vi "Test_sqlite3QueriesWithNoDatabase_ReturnsError.vi"(8 "error in (no error)":errorcluster, 11 "TestCase in":refnum<class "Test sqlite3.lvclass">) -> (0 "error out":errorcluster, 3 "TestCase out":refnum<class "Test sqlite3.lvclass">)   [LabVIEW 2020, in "Test sqlite3.lvclass"]
uses:
  Test sqlite3.lvclass
  externals/sqlite3/Source/sqlite3.lvclass
  09da7179-2a0d-49b1-a176-e0431276ce58.vi
  <vilib>/Utility/error.llb/Error Cluster From Error Code.vi
  <vilib>/addons/_JKI Toolkits/VI Tester/TestCase.llb/TestCase.lvclass
  externals/database-interface/IDatabase/IDatabase/IDatabase.lvclass
  C:/Program Files/National Instruments/LabVIEW 2020/vi.lib/addons/_JKI Toolkits/VI Tester/TestCase.llb/TestCase.lvclass
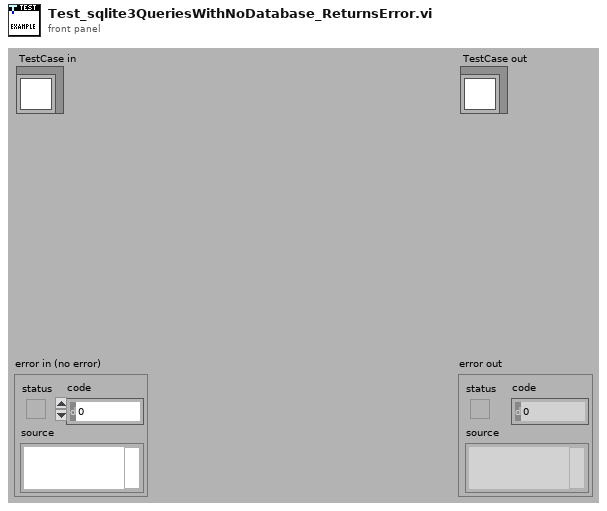
[diagram p1: front panel]
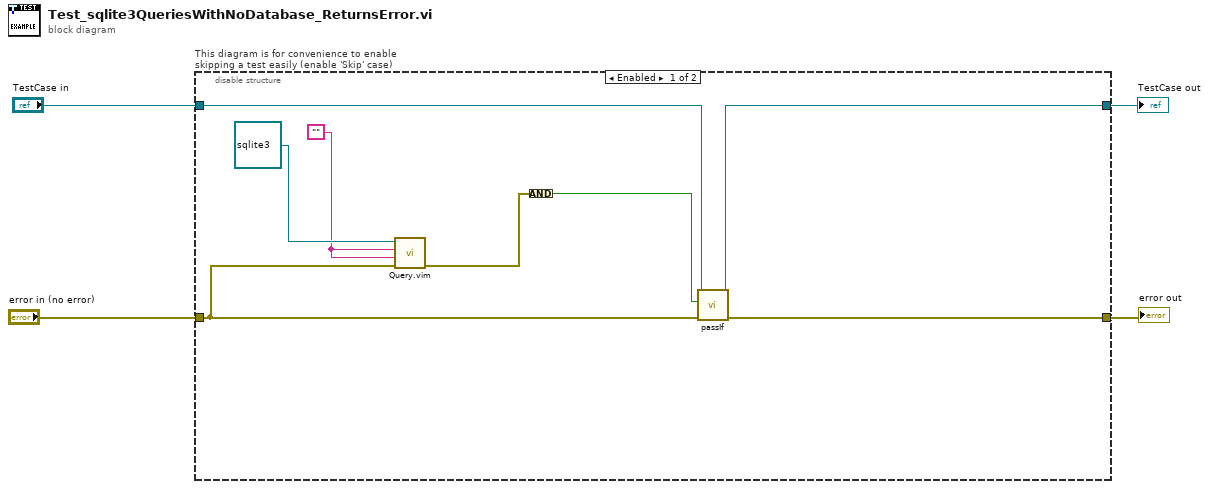
[diagram p0: block diagram]
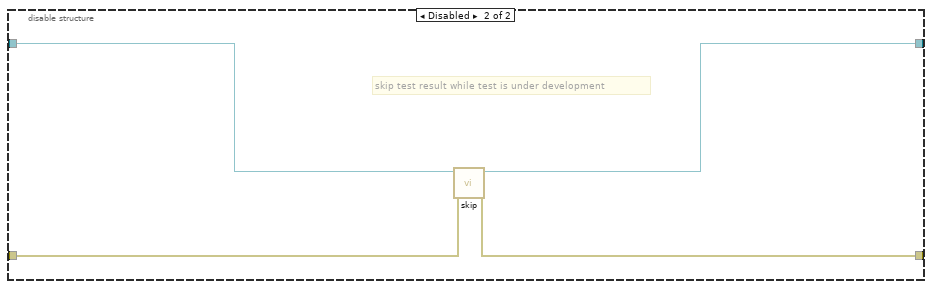
[diagram p2: hidden frame]
diagram:
  n1 = disable-structure "This diagram is for convenience to enable skipping a test easily (enable 'Skip' case)" shown="Enabled" {
    disable-tunnel: "TestCase in" -> [w10 w16]
    disable-tunnel: [w12 w14] -> w1
    disable-tunnel: [w11 w15] -> w3
    disable-tunnel: "error in (no error)" -> [w8 w13]
    frame Enabled {
      w5 = ""
      n2 = call "Query.vim"("error in (no error)"=w8, "Type and Default"=w5, "Query string"=w5, "IDatabase in"=refnum<class "sqlite3.lvclass"> refnum ("sqlite in")) -> ("error out"=w9:errorcluster)  [unwired: 5 in, 2 out]
      n3 = Compound Arithmetic op=AND(w9) -> (w6:bool)
      n4 = call-dynamic "passIf.vi"("error in (no error)"=w8, "pass"=w6, "TestCase in"=w10) -> ("error out"=w11:errorcluster, "TestCase out"=w12:refnum<class "Test sqlite3.lvclass">)  [unwired: 7 in]
    }
    frame Disabled {
      # "skip test result while test is under development"
      n5 = call <vilib>:"skip.vi"("error in (no error)"=w13, "TestCase in"=w16) -> ("error out"=w15:errorcluster, "TestCase out"=w14:refnum<class "Test sqlite3.lvclass">)  [unwired: 8 in]
    }
  }
  "error out" <- w3
  "TestCase out" <- w1
